vi "gRPC Client Test.vi"() -> ()   [LabVIEW 2023, in "Generated_client.lvlib"]
doc: "Test gRPC Service"
uses:
  Generated_client.lvlib
  RPC Messages/HelloRequest.ctl
  RPC Messages/HelloReply.ctl
panel:
  in  "gRPC Server address":string
  out "Response Data":T1
  in  "Request Data":T2
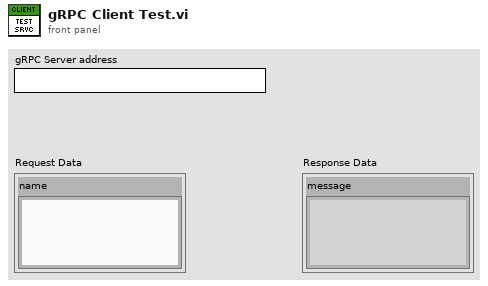
[diagram p1: front panel]
types:
  T1 = typedef "Generated_client.lvlib/HelloReply.ctl" = cluster{"message":string}
  T2 = typedef "Generated_client.lvlib/HelloRequest.ctl" = cluster{"name":string}
  T3 = typedef "grpc-lvsupport-release.lvlib/grpcId.ctl" = u64
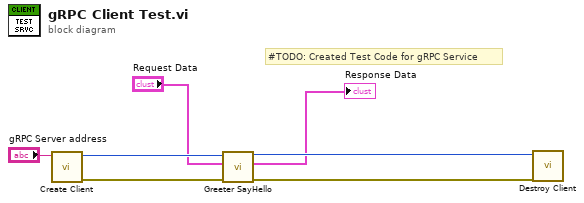
[diagram p0: block diagram]
diagram:
  # "#TODO: Created Test Code for gRPC Service"
  n1 = call "Create Client.vi"("address"="gRPC Server address") -> ("error out"=w4:errorcluster, "gRPC ID Out"=w7:T3)  [unwired: 9 in]
  n2 = call "Greeter SayHello.vi"("error in"=w4, "Request Data"="Request Data", "gRPC ID"=w7) -> ("error out"=w3:errorcluster, "Response Data"=→"Response Data":T1, "gRPC ID out"=w6:T3)  [unwired: 6 in]
  n3 = call "Destroy Client.vi"("error in"=w3, "gRPC ID"=w6) -> ()  [unwired: 9 in, 1 out]
